vi "NIDCPower_channel_ganging - measure multiple.vi"(8 "error in (no error)":errorcluster, 10 "count (1)":i32=1, 11 "Ganged Session In":T1) -> (0 "error out":errorcluster, 1 "current measurements":dbl[](array[numeric]) caption="channel current measurements", 2 "voltage measurements":dbl[](array[numeric]), 3 "Ganged Session Out":T1, 4 "Some Channels in compliance?":bool, 5 "ganged current measurement":dbl, 6 "All Channels in compliance?":bool, 7 "ganged voltage measurement":dbl)   [LabVIEW 2021]
uses:
  ctl/NIDCPower_channel_ganging - ctl - ganged session.ctl
  ctl/NIDCPower_channel_ganging - ctl - ganged config.ctl
  ctl/NIDCPower_channel_ganging - ctl - channel mode.ctl
  <instrlib>/niDCPower/nidcpower.llb/niDCPower Send Software Edge Trigger - Signal.ctl
  <vilib>/Analysis/baseanly.llb/Mean (DBL).vi
  <vilib>/Analysis/NI_AALBase.lvlib
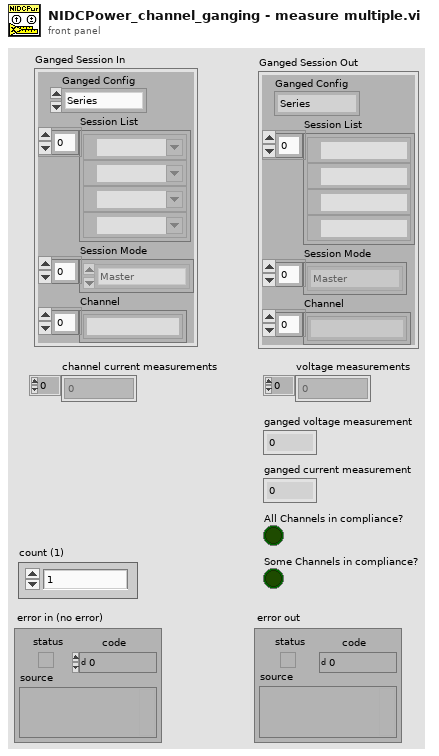
[diagram p1: front panel]
types:
  T1 = typedef "NIDCPower_channel_ganging - ctl - ganged session.ctl" = cluster{"Ganged Config":T2, "Session List":refnum<k15>[], "Session Mode":T3[], "Channel":string[]}
  T2 = typedef "NIDCPower_channel_ganging - ctl - ganged config.ctl" = enum32{"Series", "Parallel", "Manual"}
  T3 = typedef "NIDCPower_channel_ganging - ctl - channel mode.ctl" = enum32{"Master", "Slave", "Slave - Inverted"}
  T4 = typedef "niDCPower Send Software Edge Trigger - Signal.ctl" = i32
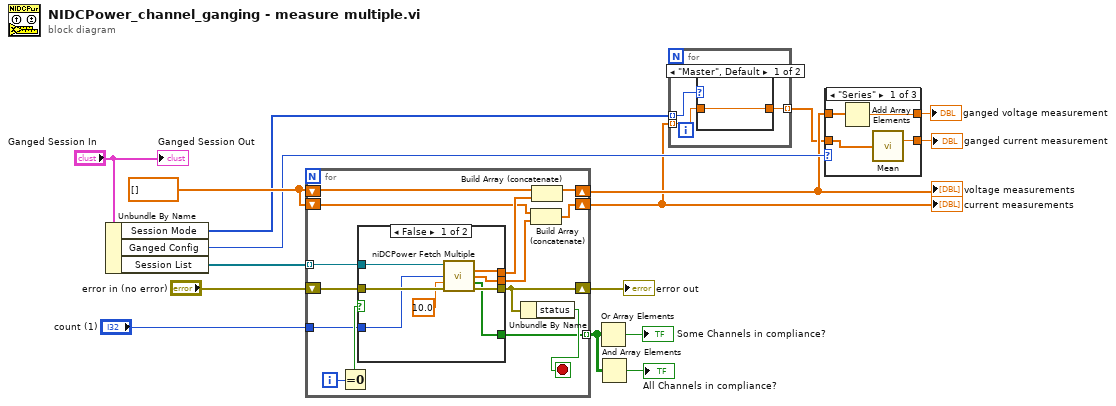
[diagram p0: block diagram]
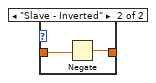
[diagram p2: hidden frame]
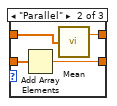
[diagram p3: hidden frame]
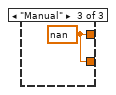
[diagram p4: hidden frame]
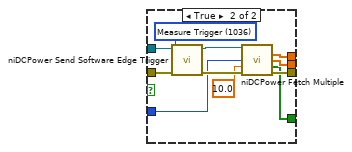
[diagram p5: hidden frame]
diagram:
  w14 = dbl[] [] ("voltage measurements")
  n1 = Unbundle By Name("Ganged Session In") -> ("Session Mode"=w2:T3[], "Ganged Config"=w10:T2, "Session List"=w12:refnum<k15>[])
  n2 = for {
    shift-right: [w20] -> w15
    shift-left: "error in (no error)" -> [w30]
    tunnel: w12 -> [w29] mode=indexing
    shift-right: [w26] -> w9
    shift-left: w14 -> [w28]
    shift-right: [w23] -> w4
    shift-left: w14 -> [w25]
    tunnel: [w18] -> w5 mode=indexing
    tunnel: "count (1)" -> [w17]
    i -> [w22]
    stop <- w19 stop-if-true
    n3 = Equal To 0?(x=w22) -> (x = 0?=w21:bool)
    n4 = case shown="False" w21 {
      tunnel: w30 -> [w38 w45]
      tunnel: w29 -> [w37 w46]
      tunnel: [w36 w49] -> w20
      tunnel: [w35 w48] -> w27
      tunnel: [w34 w47] -> w24
      tunnel: [w33 w41] -> w18
      tunnel: w17 -> [w32 w40]
      frame False {
        n5 = call <instrlib>:"niDCPower Fetch Multiple.vi"("instrument handle"=w37, "count (1)"=w32, "timeout (1.0)"=10.0, "error in (no error)"=w38) -> ("voltage measurements"=w35:dbl[], "current measurements"=w34:dbl[], "in compliance"=w33:bool[], "error out"=w36:errorcluster)  [unwired: 6 in, 2 out]
      }
      frame True {
        w42 = T4 1036 items=["Start Trigger"=1034, "Source Trigger"=1035, "Measure Trigger"=1036, "Sequence Advance Trigger"=1037] ("signal")
        n6 = call <instrlib>:"niDCPower Send Software Edge Trigger.vi"("error in (no error)"=w45, "signal"=w42, "instrument handle"=w46) -> ("error out"=w44:errorcluster, "instrument handle out"=w43:refnum<k15>)  [unwired: 7 in]
        n7 = call <instrlib>:"niDCPower Fetch Multiple.vi"("instrument handle"=w43, "count (1)"=w40, "timeout (1.0)"=10.0, "error in (no error)"=w44) -> ("voltage measurements"=w48:dbl[], "current measurements"=w47:dbl[], "in compliance"=w41:bool[], "error out"=w49:errorcluster)  [unwired: 6 in, 2 out]
      }
    }
    n8 = Unbundle By Name(w20) -> ("status"=w19:bool)
    n9 = Build Array (concatenate)(w25, w24) -> (w23:dbl[])
    n10 = Build Array (concatenate)(w28, w27) -> (w26:dbl[])
  }
  "error out" <- w15
  "voltage measurements" <- w9
  "current measurements" <- w4
  n11 = Or Array Elements(Boolean array=w5) -> (logical OR=→"Some Channels in compliance?":bool)
  n12 = And Array Elements(Boolean array=w5) -> (logical AND=→"All Channels in compliance?":bool)
  n13 = for {
    tunnel: w2 -> [w52] mode=indexing
    tunnel: w4 -> [w51] mode=indexing
    tunnel: [w50] -> w3 mode=indexing
    n14 = case shown="\"Master\", Default" w52 {
      tunnel: [w53 w55] -> w50
      tunnel: w51 -> [w53 w54]
      frame "Master", Default {
      }
      frame "Slave - Inverted" {
        n15 = Negate(x=w54) -> (-x=w55:dbl)
      }
    }
  }
  n16 = case shown="\"Series\"" w10 {
    tunnel: w9 -> [w59 w61 _]
    tunnel: w3 -> [w57 w63 _]
    tunnel: [w56 w62 w64] -> w7
    tunnel: [w58 w60 w64] -> w8
    frame "Series" {
      n17 = Add Array Elements(numeric array=w59) -> (sum=w58:dbl)
      n18 = call-poly <vilib>:"Mean.vi"("X"=w57) -> ("mean"=w56:dbl)  [unwired: 1 out]
    }
    frame "Parallel" {
      n19 = Add Array Elements(numeric array=w63) -> (sum=w62:dbl)
      n20 = call-poly <vilib>:"Mean.vi"("X"=w61) -> ("mean"=w60:dbl)  [unwired: 1 out]
    }
    frame "Manual" {
      w64 = nan
    }
  }
  "ganged voltage measurement" <- w8
  "ganged current measurement" <- w7
  "Ganged Session Out" <- "Ganged Session In"
